vi "Set target torque.vi"(6 "Torque":i16(knob) scale=-200.0..200.0, 7 "timeout (1s)":dbl=1.0 min=0.0, 8 "error in (no error)":errorcluster, 11 "SDO object in":refnum<k20>) -> (0 "error out":errorcluster, 1 "completion code":u32, 3 "SDO object out":refnum<k20>)   [LabVIEW 2016]
uses:
  <vilib>/CANopenLib/CANOPEN.llb/CANopen SDO Write [I16].vi
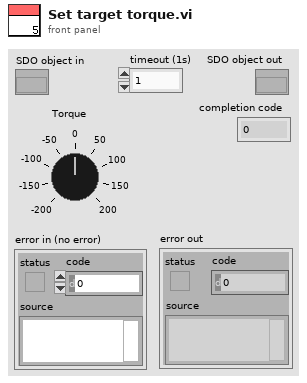
[diagram p1: front panel]
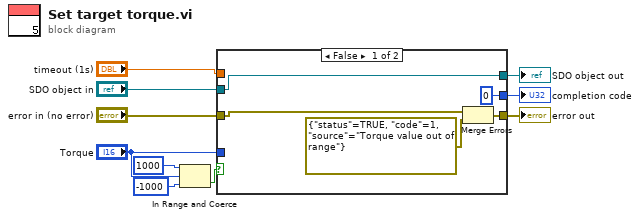
[diagram p0: block diagram]
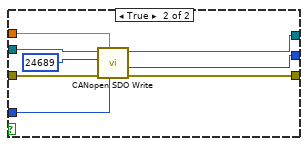
[diagram p2: hidden frame]
diagram:
  n1 = In Range and Coerce(upper limit=i16 1000, x="Torque", lower limit=i16 -1000) -> (In Range?=w4:bool)  [unwired: 1 out]
  n2 = case shown="False" w4 {
    tunnel: [u32 0 ("completion code") w23] -> w10
    tunnel: "Torque" -> [_ w21]
    tunnel: [w15 w20] -> w9
    tunnel: "error in (no error)" -> [w13 w19]
    tunnel: "timeout (1s)" -> [_ w18]
    tunnel: "SDO object in" -> [w11 w17]
    tunnel: [w11 w16] -> w5
    frame False {
      n3 = Merge Errors(w13, errorcluster {"status"=TRUE, "code"=1, "source"="Torque value out of range"} ("error constant")) -> (w15:errorcluster)
    }
    frame True {
      n4 = call-poly <vilib>:"CANopen SDO Write.vi"("I16 data"=w21, "timeout (1s)"=w18, "error in (no error)"=w19, "object index"=u16 24689, "SDO object in"=w17) -> ("error out"=w20:errorcluster, "completion code"=w23:u32, "SDO object out"=w16:refnum<k20>)  [unwired: 4 in]
    }
  }
  "completion code" <- w10
  "error out" <- w9
  "SDO object out" <- w5
